vi "Get Current Config.vi"(8 "error in":errorcluster) -> (0 "error out":errorcluster, 3 "Configuration":T1)   [LabVIEW 2020, in "Performance Monitor UI.lvlib" / "Configuration.lvclass"]
doc: "Wrapper for the private global to read the stored configuration.\n____\nPeloton Config 2.0.0.6\nCopyright (c) 2024, Peloton"
uses:
  Configuration.lvclass
  Configuration--cluster.ctl
  Configuration.lvclass/Configuration.ctl
  Get Configuration.vi
  <vilib>/Peloton/Peloton Config/DCFG Framework/Peloton_lib_DCFG Framework.lvlib
  Performance Monitor UI.lvlib
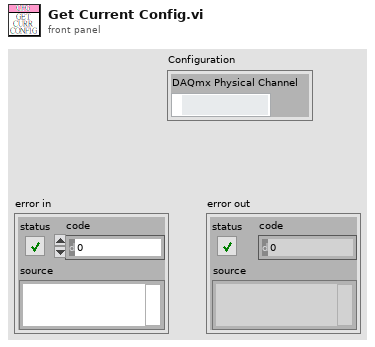
[diagram p1: front panel]
types:
  T1 = typedef "Performance Monitor UI.lvlib/Configuration.lvclass/Configuration--cluster.ctl" = cluster{"DAQmx Physical Channel":tag}
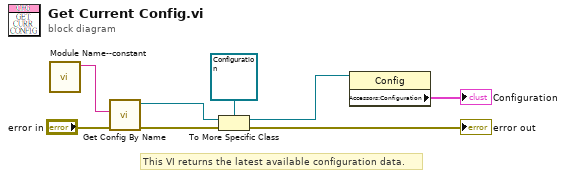
[diagram p0: block diagram]
diagram:
  # "This VI returns the latest available configuration data."
  n1 = call "Module Name--constant.vi"() -> ("Module Name"=w3:string)  [unwired: 11 in]
  n2 = call <vilib>:"Get Config By Name.vi"("error in"="error in", "Config Name"=w3) -> ("error out"=w8:errorcluster, "DCFG Framework.lvlib:Config"=w7:refnum<class "Configuration.lvclass">)  [unwired: 7 in, 1 out]
  n3 = To More Specific Class(target class=refnum<class "Configuration.lvclass"> refnum ("Sample Module 1.lvlib:Config"), reference=w7, error in=w8) -> (specific class reference=w5:refnum<class "Configuration.lvclass">, error out=→"error out":errorcluster)
  n4 = property class="Config"(reference=w5) -> ("Accessors:Configuration"=→"Configuration":T1)  [unwired: 1 in, 2 out]
